vi "GCDiode.vi"(2 "Run uninterrupted?":bool, 3 "Device Category IN:":string(combo)="ATLAS18SS" caption="Device Category:", 4 "Batch No. IN:":string caption="Batch No.:", 5 "Wafer No. IN:":string caption="Wafer No.:", 6 "DB Serial No. IN:":string caption="DB Serial No.:") -> (0 "Done!":bool)   [LabVIEW 2013]
doc: "Performs measurements on gate-controlled diodes on sensor halfmoons according to ATLAS ITk QA Specifications."
uses:
  InstrControl/SupplyControl/SupplyControl.lvclass
  general_VIs/globals/QC_MeasurementSetup.vi
  general_VIs/globals/QC_RunInformation.vi
  InstrControl/InstrumentSetup.vi
  InstrControl/ArduinoControl/ArduinoControl.lvclass
  <vilib>/Analysis/NI_AALBase.lvlib
  InstrControl/InstrControl.lvclass
panel:
  out "Tab Control 2":enum32{"GCD Setup", "GCD Scan"}(tab)
  in  "Bias voltage [V]":dbl=5.0
  in  "Set current limit?":bool
  in  "Current Limit [µA]":dbl=1000.0 min=0.0001 format="%.3f"
  in  "Measurement Configurations":bool
  in  "Initial volts [V] IN":dbl=-10.0 caption="Initial volts [V]"
  in  "Final volts [V] IN":dbl=20.0 caption="Final volts [V]"
  in  "step [V] IN":dbl=0.5 caption="step [V]" format="%.1f"
  in  "step interval [s] IN":i32=1 caption="step interval [s]"
  in  "Continue":bool
  in  "Quit":bool
  out "Bias volts [V]":dbl=5.0 format="%.1f"
  out "RH":dbl[](array[numeric]) caption="RH [%]" format="%#.2f"
  out "Temp.":dbl[](array[numeric]) caption="Temp. [°C]" format="%#.2f"
  out "Current":dbl[](array[numeric]) caption="Current [nA]"
  out "Volts":dbl[](array[numeric]) caption="Volts [V]"
  out "step interval [s]":i32=1
  out "step [V]":dbl=0.5 format="%.1f"
  out "Final volts [V]":dbl=20.0 format="%.1f"
  out "Initial volts [V]":dbl=-10.0 format="%.1f"
  out "Igraph":cluster{dbl[], dbl[]}(graph)
  in  "Scales":T1(ring)
  in  "Iscale":enum16{"nanoAmps", "microAmps", "milliAmps"}(ring)
  out "positive ramp?":bool
  out "Tab Control":enum32{"GCD Setup", "GCD Scan"}(tab)
  in  "Test SMU":string(combo)="Keithley 2410"
  in  "Hardware Configurations":bool
  in  "User:":string(combo)="Christoph"
  in  "Bias Supply":string(combo)="Keithley 6517"
  in  "Temperature":enum16{"Read Arduino", "Enter manually"}(ring)=enum."Enter manually"
  in  "Manufacturer:":string(combo)="Hamamatsu"
  in  "abort":bool
  out "Device Category:":string
  out "DB Serial No.:":string
  out "Current Volts:":dbl format="%.2f"
  in  "quit (no save)":bool
  in  "Quit & Save":bool
  out "Bias On/Off:":bool
  out "STATUS 1":string
  out "Initiated:":string
  out "Sensor No.:":string
  out "No of steps":u32
  out "Current reading No.":u32
  out "Last reading at:":string
  # "University of\nCambridge"
  # "Strip Sensor QA: Gate-controlled Diode"
  # "Vertical Scale:"
  # "Measurement Configuration"
  # "IV Scan parameters:"
  # "Last 3 readings:"
  # "n-2"
  # "n-1"
  # "n"
  # "DUT Description"
  # "Hardware"
  # "DUT & Test Description:"
  # "Current status:"
  # "Rdg No:"
  # "out of"
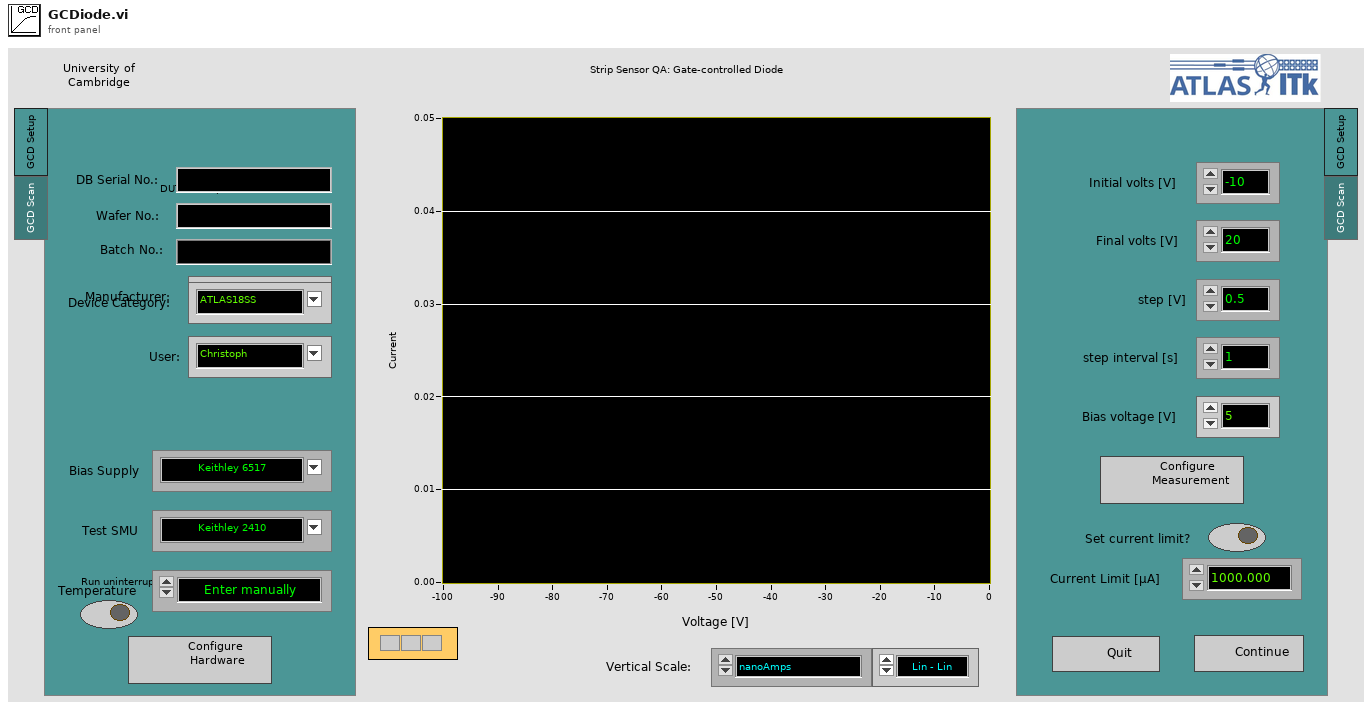
[diagram p1: front panel]
types:
  T1 = enum16{"Lin - Lin", "Log - Lin", "Lin - Log", "Log - log"}
  T2 = enum16{"Supply", "LCR", "Multimeter", "Switching"}
  T3 = enum16{"Reset", "Read Array", "Read Element", "Write Element", "Write Array", "Add Element", "Add Array"}
  T4 = cluster{"Institute":string, "Manufacturers":string[], "Devices":string[], "Serialnumbers Lookup DB":string, "Data directory":string, "Backup & screenshot directory":string, "List of known users":string[], "Measurement switch not used":bool, "Measurement Switch":string, "DUT Switch":string, "Rseries IV [MOhm]":string, "Rshunt IV [MOhm]":string, "Rseries CV [MOhm]":string, "DC blocking Cap [µF]":string, "Rseries LCR [MOhm]":string, "Rseries stability [MOhm]":string, "Rshunt stability [MOhm]":string, "Rseries striptest bias [MOhm]":string, "Rseries strip pinhole [MOhm]":string}
  T5 = cluster{"Sensor Serial No.:":string, "Wafer:":string, "Batch:":string, "Manufacturer:":string, "Device Category:":string, "Database Serial No.:":string, "Date Initiated:":string, "Time Initiated:":string, "Test":string, "Probeplan used:":string, "End of Run comment:":string, "User:":string, "Vbias SMU":string, "LCR":string, "Test SMU":string, "Test DMM":string}
  T6 = cluster{"Bias Supply":refnum<class "SupplyControl.lvclass">, "SMU":refnum<class "SupplyControl.lvclass">, "Arduino":refnum<class "ArduinoControl.lvclass">, "Initial Voltage [V]":dbl, "Final Voltage [V]":dbl, "Step Size [V]":dbl, "Step Interval [s]":i32, "Number Of Steps":u32, "Ramp down steps [V]":dbl, "Ramp down Interval [s]":i32, "Bias Voltage [V]":dbl, "Set Current Limit?":bool, "Current Limit [µA]":dbl, "Temperature Readout":enum16{"Read Arduino", "Enter manually"}, "Bias Supply Name":string, "SMU Name":string}
  T7 = cluster{"VISA address":refnum<visa-resource-name>, "T sensor":enum16{"SHT", "DS"}, "Arduino":refnum<class "ArduinoControl.lvclass">}
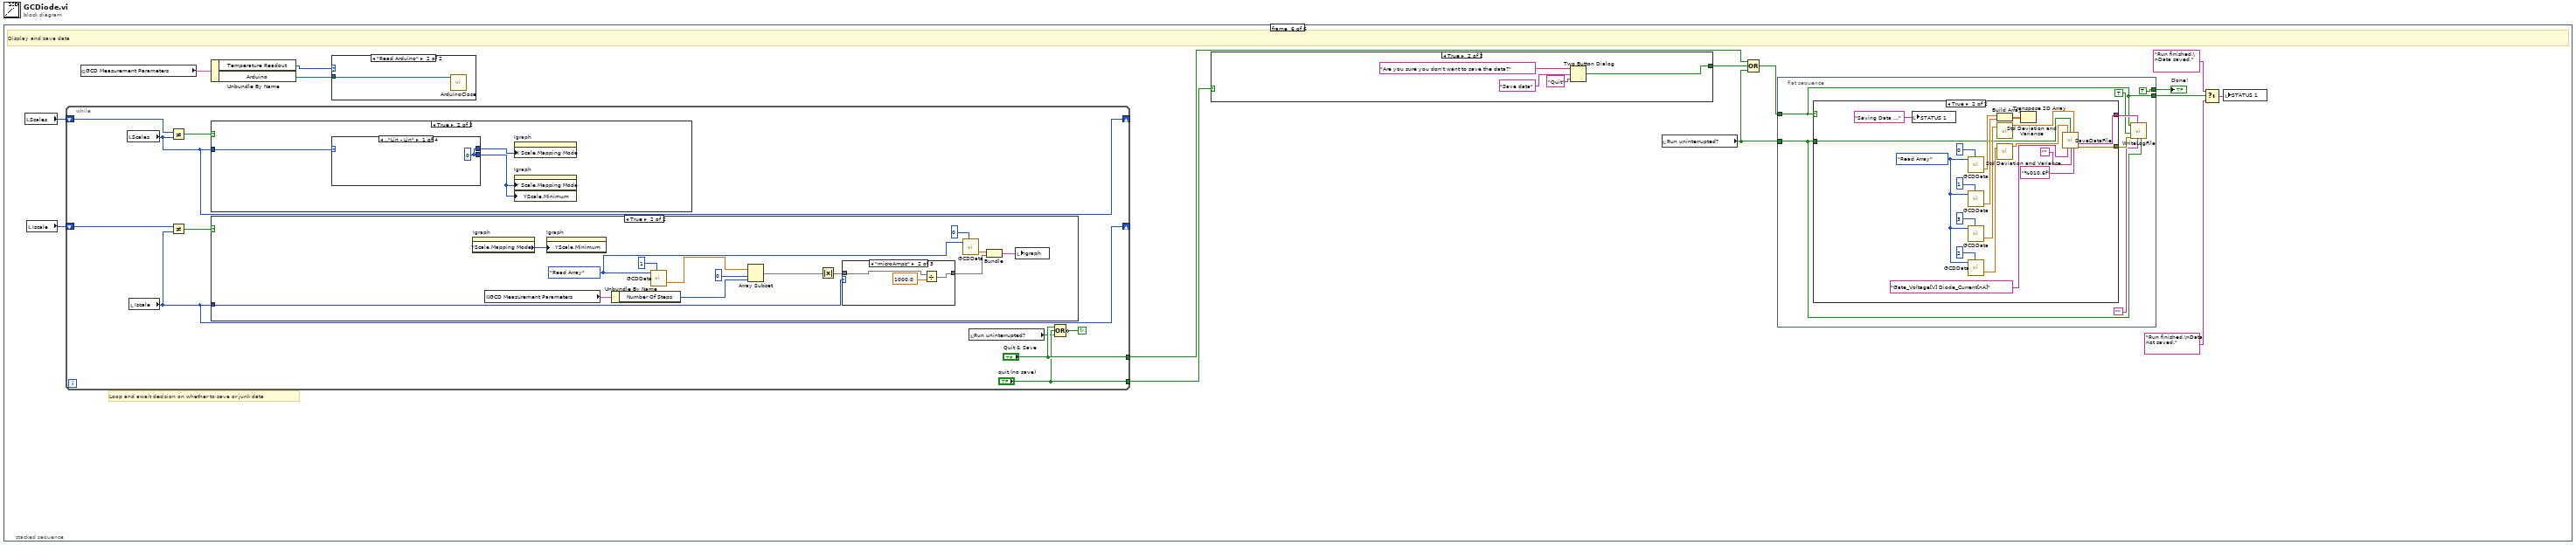
[diagram p0: block diagram]
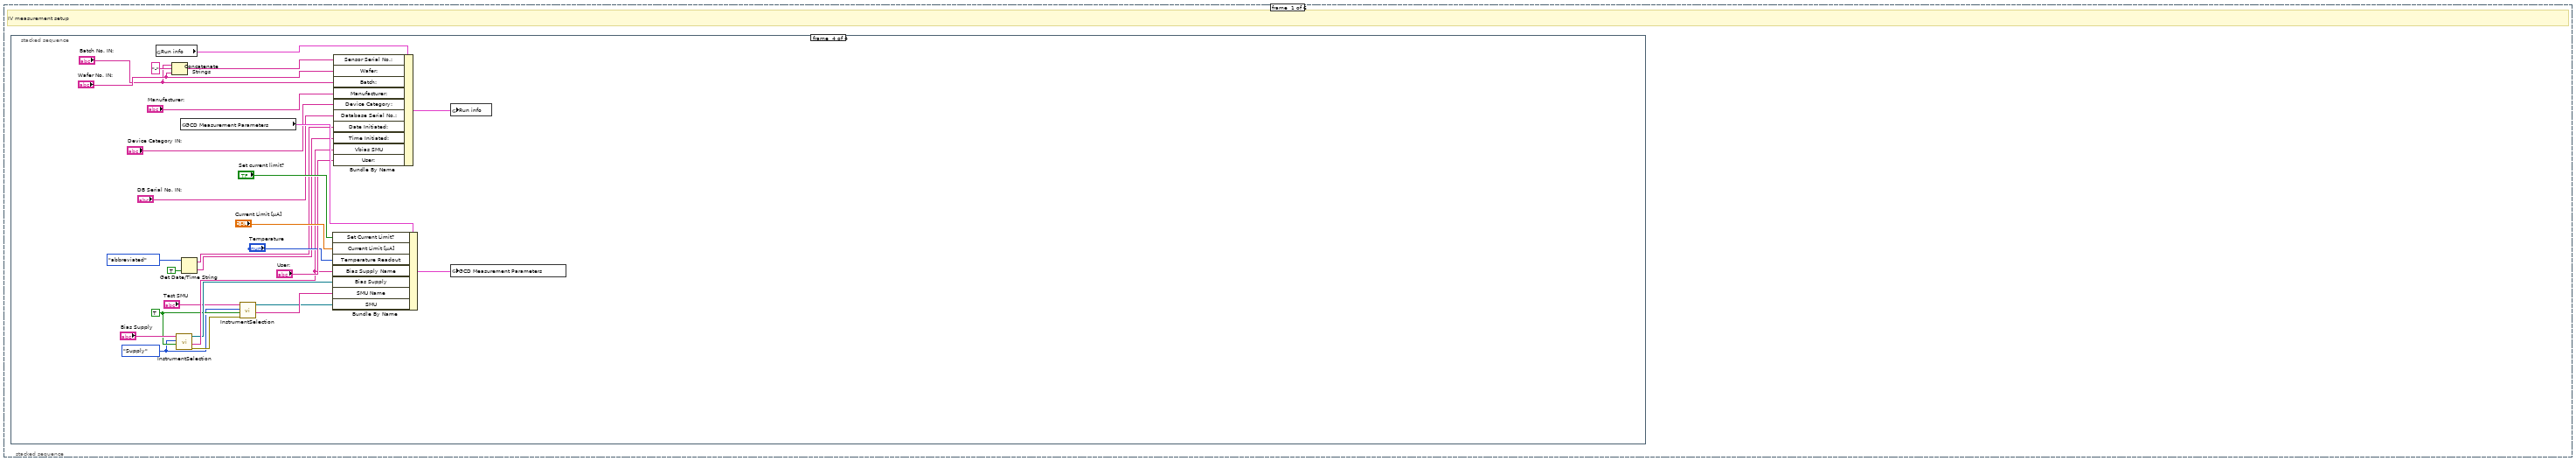
[diagram p2: hidden frame]
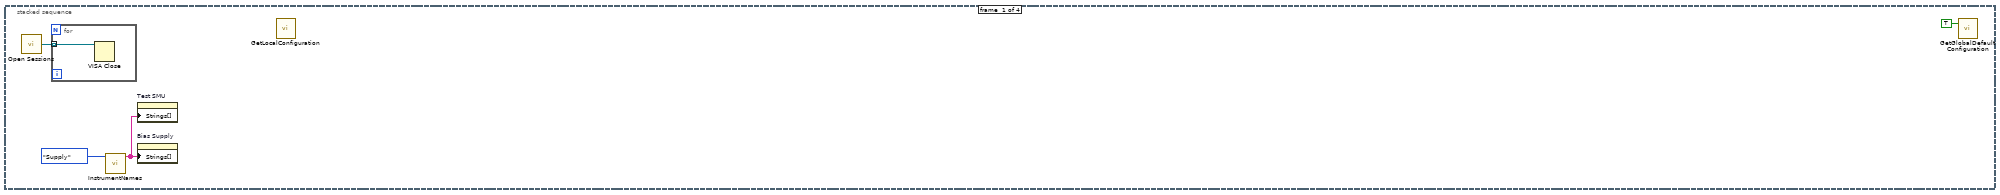
[diagram p3: hidden frame]
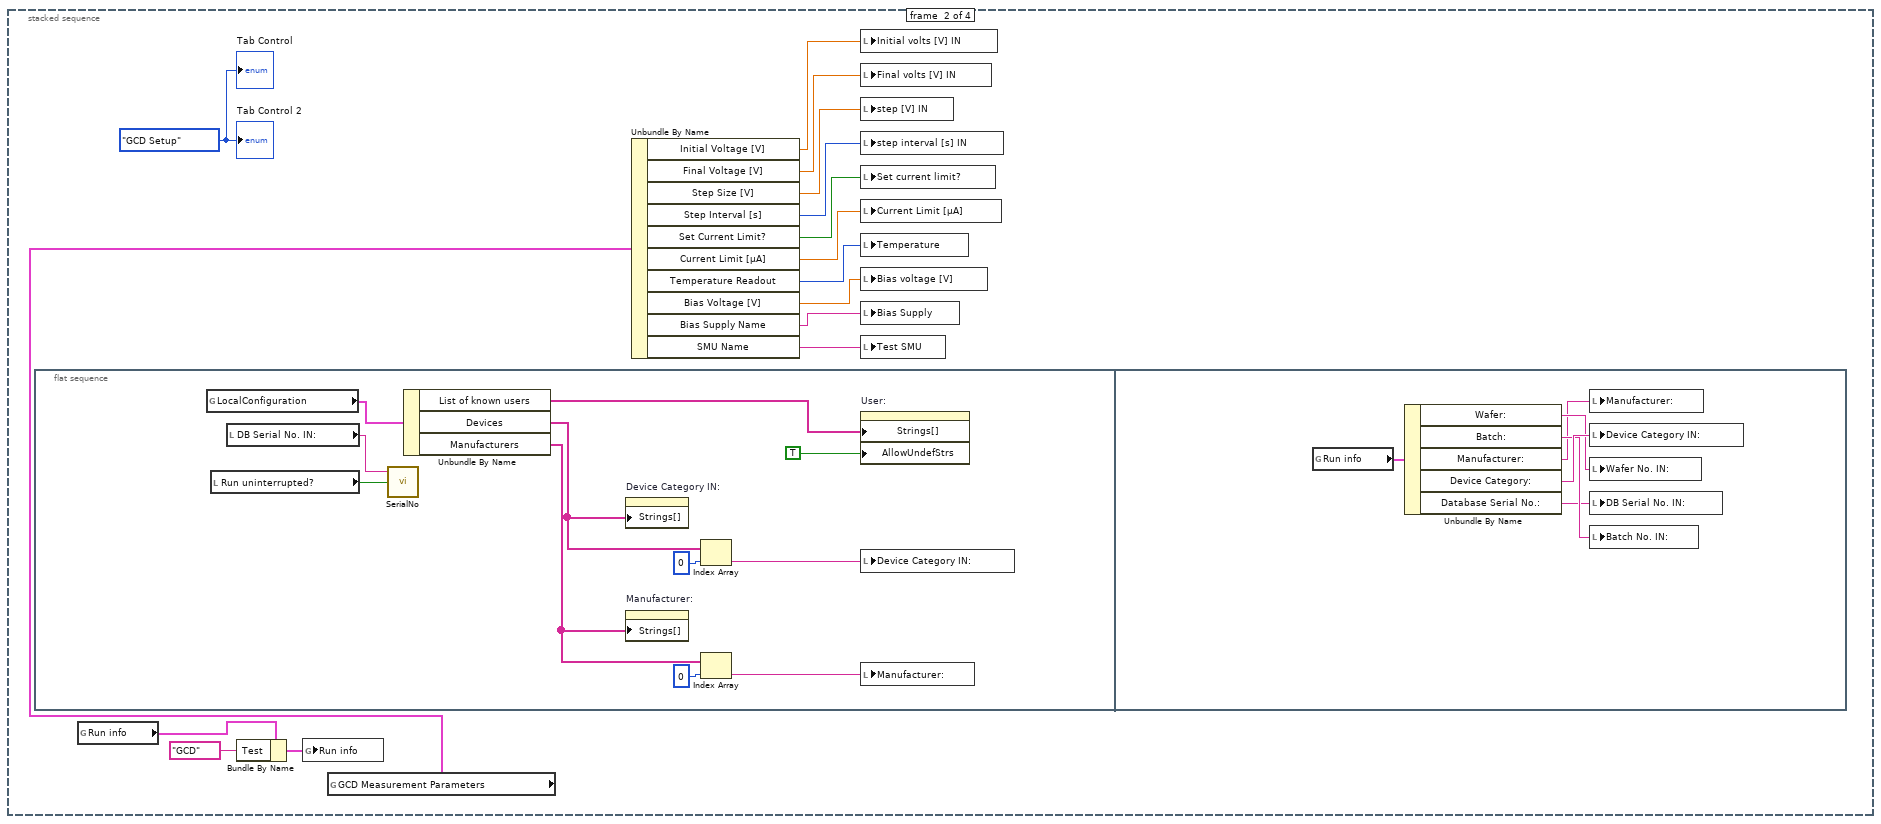
[diagram p4: hidden frame]
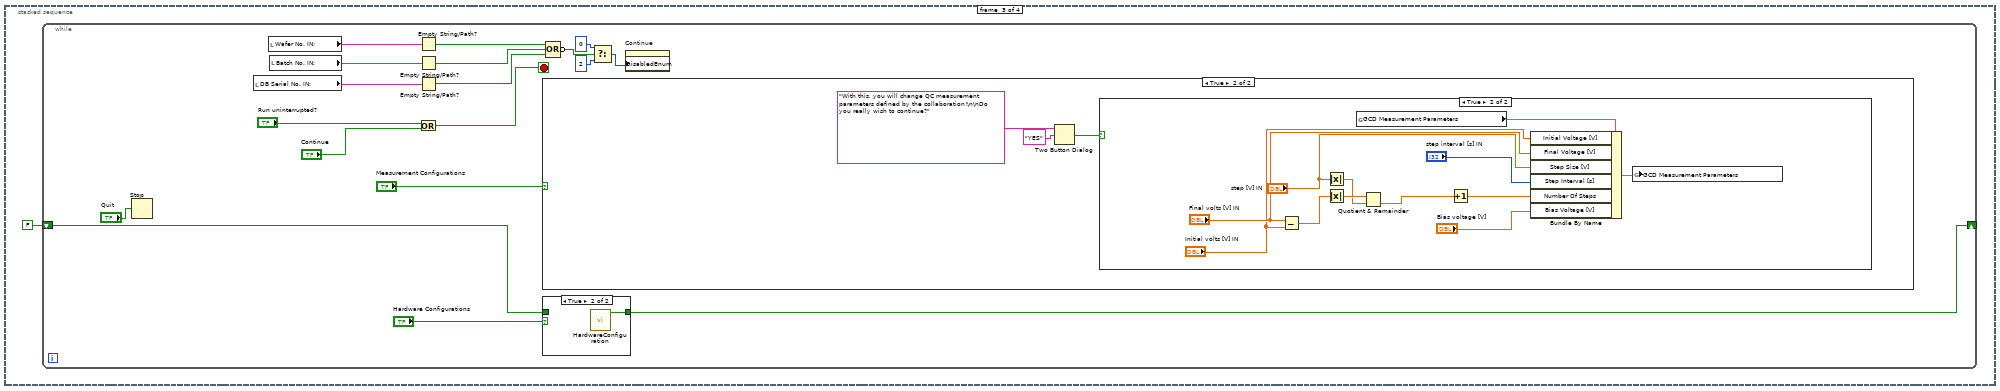
[diagram p5: hidden frame]
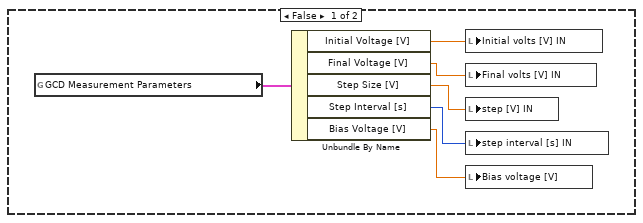
[diagram p7: hidden frame]
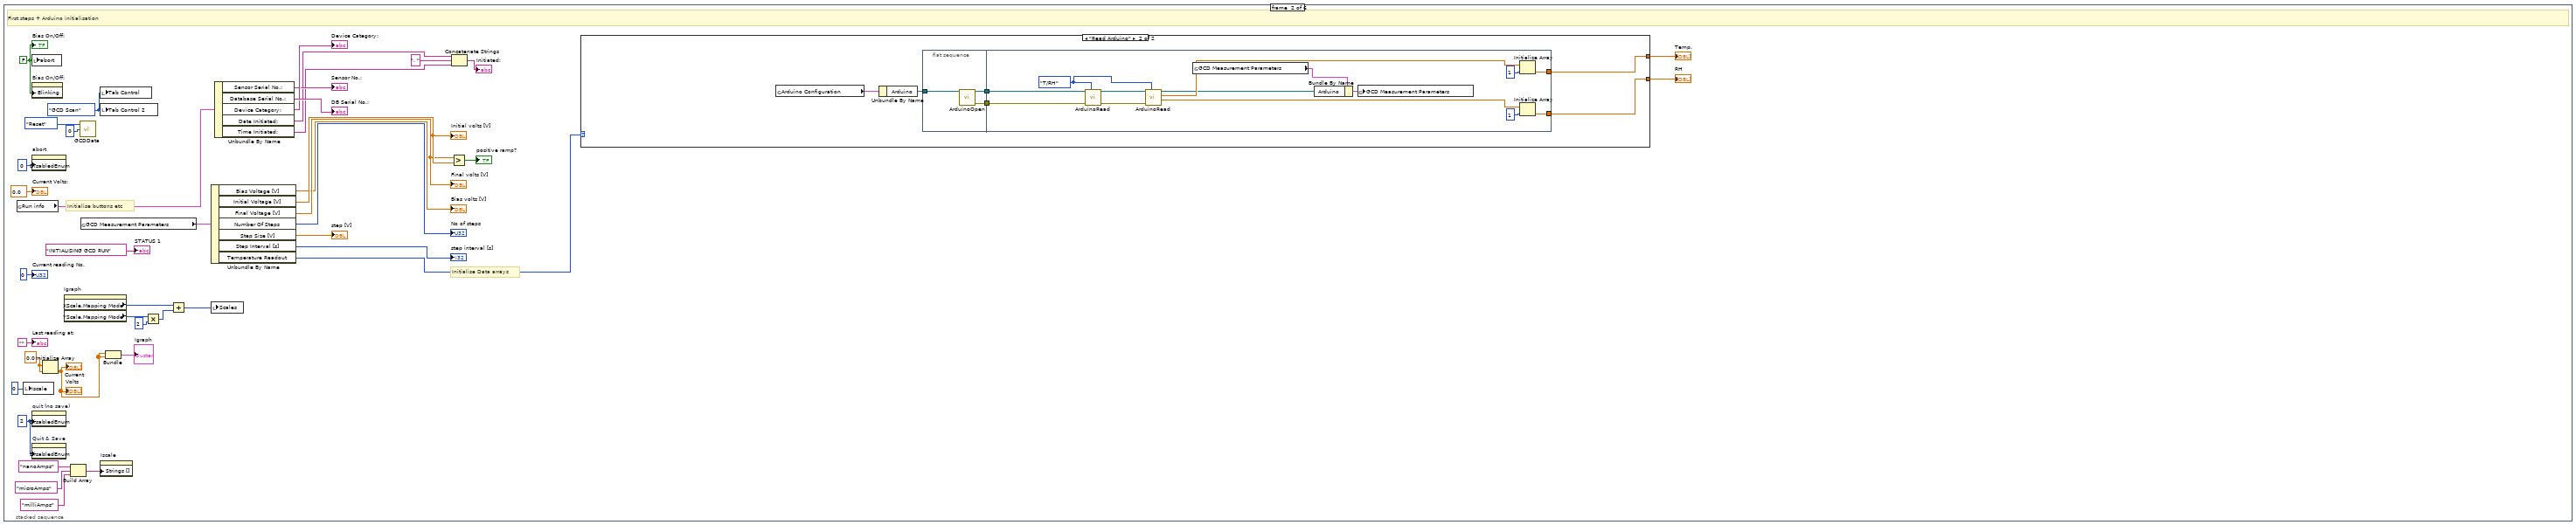
[diagram p9: hidden frame]
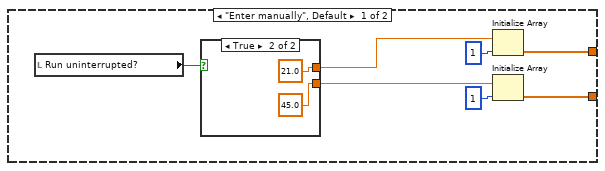
[diagram p10: hidden frame]
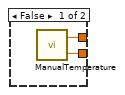
[diagram p11: hidden frame]
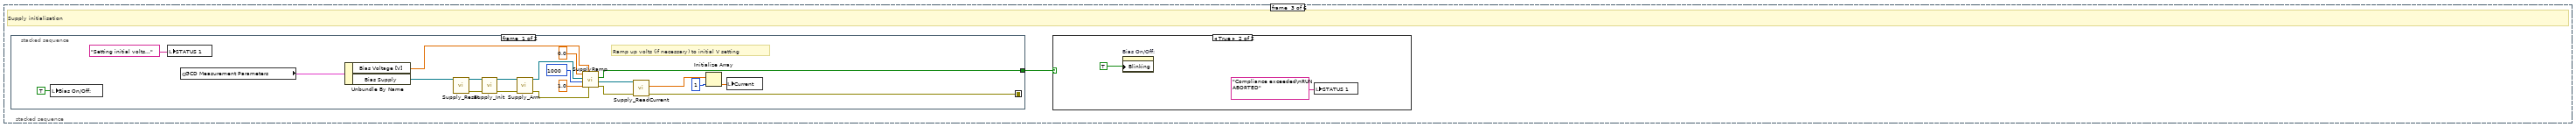
[diagram p12: hidden frame]
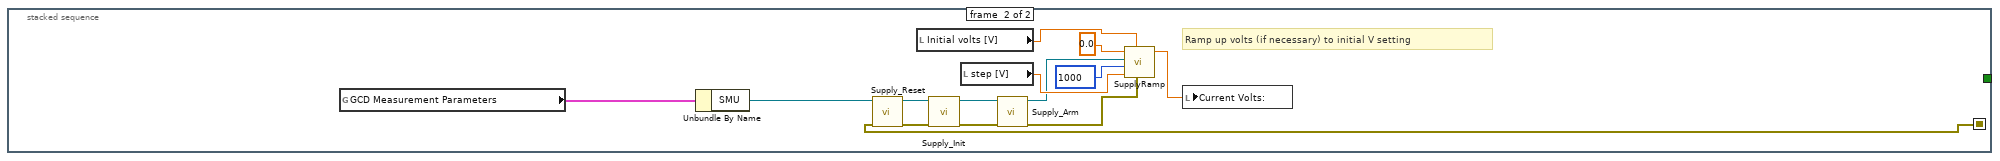
[diagram p13: hidden frame]
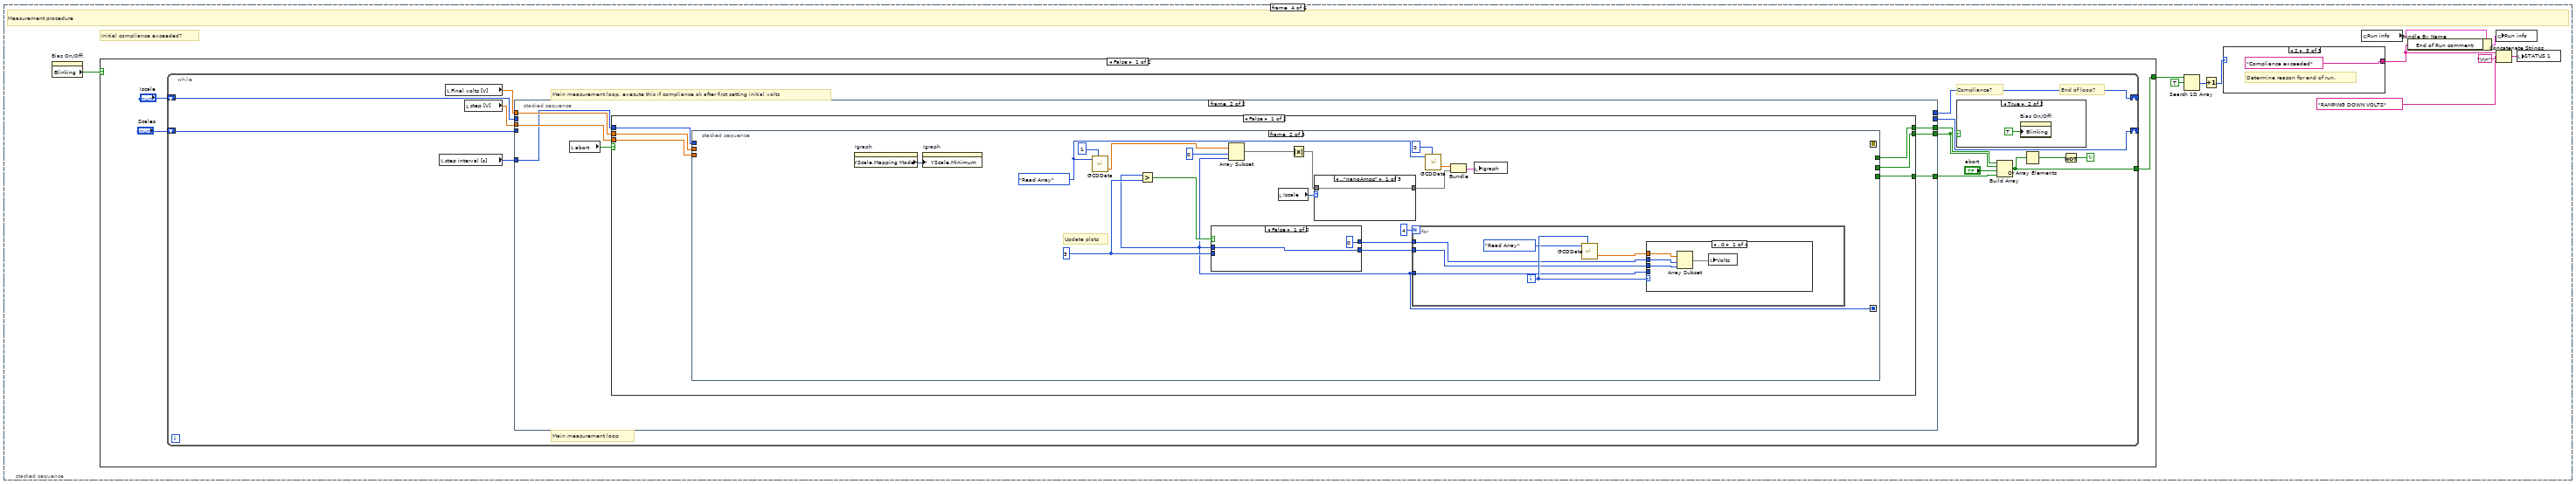
[diagram p15: hidden frame]
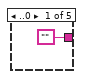
[diagram p16: hidden frame]
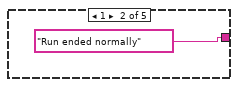
[diagram p17: hidden frame]
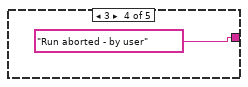
[diagram p18: hidden frame]
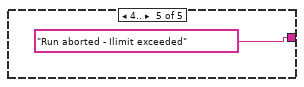
[diagram p19: hidden frame]
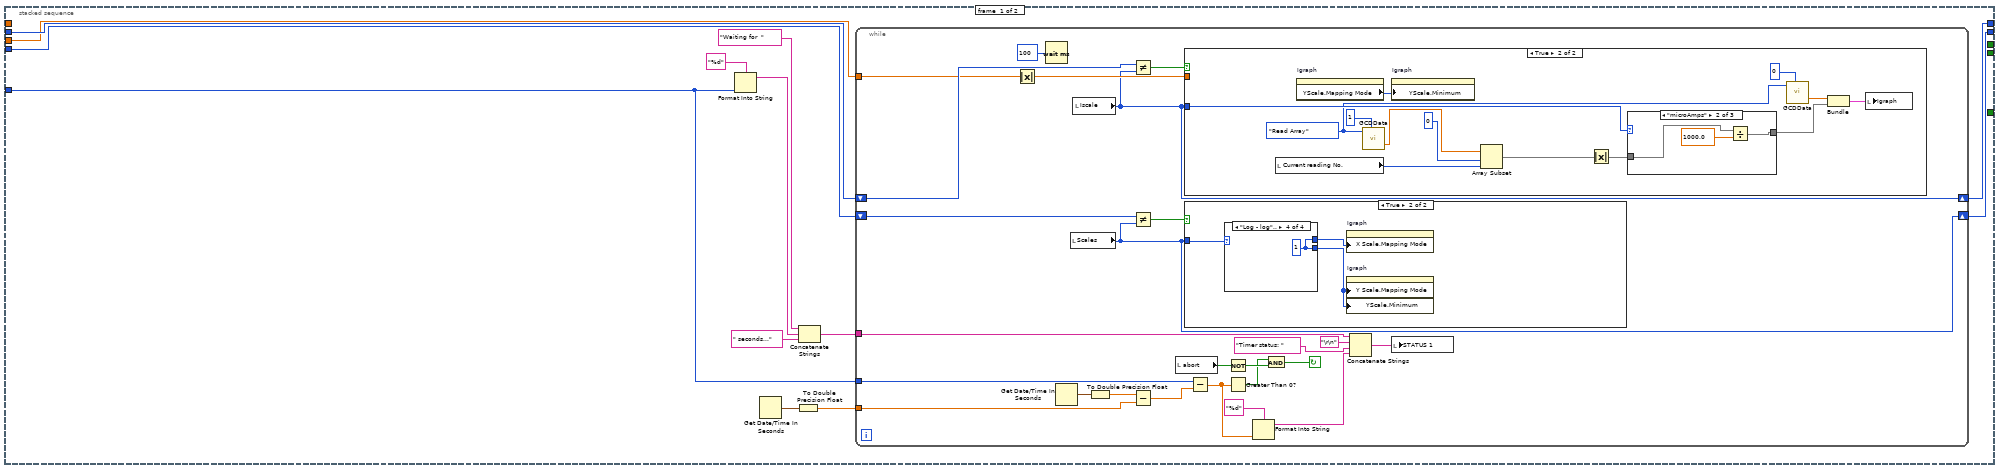
[diagram p20: hidden frame]
diagram:
  n1 = stacked-sequence {
    frame #0 {
      # "IV measurement setup"
      n2 = stacked-sequence {
        frame #0 {
          n3 = call <vilib>:"Open Sessions.vi"() -> ("Array of Refnums"=w2:refnum<visa-resource-name>[])  [unwired: 2 in]
          n4 = for {
            tunnel: w2 -> [w5] mode=indexing
            n5 = VISA Close(VISA resource name=w5) -> ()  [unwired: 1 in, 1 out]
          }
          n6 = call "InstrumentNames.vi"("Instrument type"=T2."Supply") -> ("Instrument names"=w1:string[])  [unwired: 9 in, 1 out]
          n7 = property on="Test SMU" class="CmbBox"("Strings[]"=w1) -> ()  [unwired: 2 in, 2 out]
          n8 = property on="Bias Supply" class="CmbBox"("Strings[]"=w1) -> ()  [unwired: 2 in, 2 out]
          n9 = call "GetLocalConfiguration.vi"() -> ()  [unwired: 3 in, 1 out]
          n10 = call "GetGlobalDefaultConfiguration.vi"("Read defaults?"=TRUE) -> ()  [unwired: 3 in]
        }
        frame #1 {
          w9 = enum32{"GCD Setup", "GCD Scan"}."GCD Setup" ("Tab Control")
          n11 = flat-sequence {
            frame #0 {
              n12 = global read "QC_RunInformation.vi" "LocalConfiguration"() -> (w23:T4)
              n13 = local read "Run uninterrupted?"() -> (w22:bool)
              n14 = local read "DB Serial No. IN:"() -> (w21:string)
              n15 = call "SerialNo.vi"("DB serial number IN"=w21, "Run uninterrupted?"=w22) -> ()  [unwired: 6 in, 2 out]
              n16 = Unbundle By Name(w23) -> ("List of known users"=w24:string[], "Devices"=w27:string[], "Manufacturers"=w29:string[])
              n17 = property on="Device Category IN:" class="CmbBox"("Strings[]"=w27) -> ()  [unwired: 2 in, 2 out]
              n18 = property on="Manufacturer:" class="CmbBox"("Strings[]"=w29) -> ()  [unwired: 2 in, 2 out]
              n19 = Index Array(array=w27, index=0) -> (element=w31:string)
              n20 = Index Array(array=w29, index=0) -> (element=w30:string)
              n21 = property on="User:" class="CmbBox"("Strings[]"=w24, "AllowUndefStrs"=TRUE) -> ()  [unwired: 2 in, 2 out]
              n22 = local write "Device Category IN:"(w31) -> ()
              n23 = local write "Manufacturer:"(w30) -> ()
            }
            frame #1 {
              n24 = global read "QC_RunInformation.vi" "Run info"() -> (w32:T5)
              n25 = Unbundle By Name(w32) -> ("Wafer:"=w36:string, "Batch:"=w35:string, "Manufacturer:"=w34:string, "Device Category:"=w37:string, "Database Serial No.:"=w33:string)
              n26 = local write "Manufacturer:"(w34) -> ()
              n27 = local write "Device Category IN:"(w37) -> ()
              n28 = local write "Wafer No. IN:"(w36) -> ()
              n29 = local write "DB Serial No. IN:"(w33) -> ()
              n30 = local write "Batch No. IN:"(w35) -> ()
            }
          }
          n31 = global read "QC_RunInformation.vi" "Run info"() -> (w16:T5)
          n32 = Bundle By Name(cluster=w16, "Test"="GCD") -> (w15:T5)
          n33 = global write "QC_RunInformation.vi" "Run info"(w15) -> ()
          n34 = global read "QC_MeasurementSetup.vi" "GCD Measurement Parameters"() -> (w19:T6)
          n35 = Unbundle By Name(w19) -> ("Initial Voltage [V]"=w13:dbl, "Final Voltage [V]"=w12:dbl, "Step Size [V]"=w11:dbl, "Step Interval [s]"=w14:i32, "Set Current Limit?"=w18:bool, "Current Limit [µA]"=w17:dbl, "Temperature Readout"=w20:enum16{"Read Arduino", "Enter manually"}, "Bias Voltage [V]"=w10:dbl, "Bias Supply Name"=w7:string, "SMU Name"=w6:string)
          n36 = local write "Initial volts [V] IN"(w13) -> ()
          n37 = local write "Final volts [V] IN"(w12) -> ()
          n38 = local write "step [V] IN"(w11) -> ()
          n39 = local write "step interval [s] IN"(w14) -> ()
          n40 = local write "Set current limit?"(w18) -> ()
          n41 = local write "Current Limit [µA]"(w17) -> ()
          n42 = local write "Temperature"(w20) -> ()
          n43 = local write "Bias voltage [V]"(w10) -> ()
          n44 = local write "Bias Supply"(w7) -> ()
          n45 = local write "Test SMU"(w6) -> ()
          "Tab Control" <- w9
          "Tab Control 2" <- w9
        }
        frame #2 {
          n46 = while {
            shift-right: [w46] -> _
            shift-left: FALSE -> [w45]
            stop <- w42 stop-if-true
            n47 = Stop(stop? (T)="Quit") -> ()
            n48 = local read "DB Serial No. IN:"() -> (w40:string)
            n49 = local read "Wafer No. IN:"() -> (w55:string)
            n50 = local read "Batch No. IN:"() -> (w48:string)
            n51 = Empty String/Path?(string/path=w55) -> (empty?=w54:bool)
            n52 = Empty String/Path?(string/path=w48) -> (empty?=w47:bool)
            n53 = Empty String/Path?(string/path=w40) -> (empty?=w39:bool)
            n54 = Or(x="Run uninterrupted?", y="Continue") -> (x .or. y?=w42:bool)
            n55 = case shown="True" "Measurement Configurations" {
              frame False {
              }
              frame True {
                n56 = Two Button Dialog(message="With this, you will change QC measurement parameters defined by the collaboration!\n\nDo you really wish to continue?", 2:"YES") -> (T button?=w57:bool)  [unwired: 1 in]
                n57 = case shown="True" w57 {
                  frame False {
                    n58 = global read "QC_MeasurementSetup.vi" "GCD Measurement Parameters"() -> (w65:T6)
                    n59 = Unbundle By Name(w65) -> ("Initial Voltage [V]"=w63:dbl, "Final Voltage [V]"=w64:dbl, "Step Size [V]"=w62:dbl, "Step Interval [s]"=w61:i32, "Bias Voltage [V]"=w60:dbl)
                    n60 = local write "Initial volts [V] IN"(w63) -> ()
                    n61 = local write "Final volts [V] IN"(w64) -> ()
                    n62 = local write "step [V] IN"(w62) -> ()
                    n63 = local write "step interval [s] IN"(w61) -> ()
                    n64 = local write "Bias voltage [V]"(w60) -> ()
                  }
                  frame True {
                    n65 = Subtract(x="Final volts [V] IN", y="Initial volts [V] IN") -> (x-y=w71:dbl)
                    n66 = Absolute Value(x="step [V] IN") -> (abs(x)=w72:dbl)
                    n67 = Absolute Value(x=w71) -> (abs(x)=w73:dbl)
                    n68 = global read "QC_MeasurementSetup.vi" "GCD Measurement Parameters"() -> (w77:T6)
                    n69 = Quotient & Remainder(x=w73, y=w72) -> (floor(x/y)=w69:dbl)  [unwired: 1 out]
                    n70 = Increment(x=w69) -> (x+1=w68:dbl)
                    n71 = Bundle By Name(cluster=w77, "Initial Voltage [V]"="Initial volts [V] IN", "Final Voltage [V]"="Final volts [V] IN", "Step Size [V]"="step [V] IN", "Step Interval [s]"="step interval [s] IN", "Number Of Steps"=w68, "Bias Voltage [V]"="Bias voltage [V]") -> (w74:T6)
                    n72 = global write "QC_MeasurementSetup.vi" "GCD Measurement Parameters"(w74) -> ()
                  }
                }
              }
            }
            n73 = case shown="True" "Hardware Configurations" {
              tunnel: [w78 w79] -> w46
              tunnel: w45 -> [w78 _]
              frame False {
              }
              frame True {
                n74 = call "HardwareConfiguration.vi"() -> ("configured?"=w79:bool)  [unwired: 11 in]
              }
            }
            n75 = Compound Arithmetic op=OR(w54, w47, w39) -> (invert w53:bool)
            n76 = Select(t=0, s=w53, f=2) -> (s? t:f=w50:i32)
            n77 = property on="Continue" class="Bool"("DisabledEnum"=w50) -> ()  [unwired: 2 in, 2 out]
          }
        }
        frame #3 {
          w85 = TRUE
          w80 = T2."Supply" ("Instrument type")
          n78 = global read "QC_RunInformation.vi" "Run info"() -> (w86:T5)
          n79 = Concatenate Strings("Batch No. IN:", "-", "Wafer No. IN:") -> (w87:string)
          n80 = call "InstrumentSelection.vi"("Verify GPIB address"=w85, "Instrument type"=w80, "Instrument name IN"="Bias Supply") -> ("error out"=w83:errorcluster, "Instrument name OUT"=w96:string, "Supply"=w95:refnum<class "SupplyControl.lvclass">)  [unwired: 3 in, 3 out]
          n81 = global read "QC_MeasurementSetup.vi" "GCD Measurement Parameters"() -> (w106:T6)
          n82 = Get Date/Time String(date format (0)=enum16{"short", "long", "abbreviated"}."abbreviated", want seconds? (F)=TRUE) -> (date string=w92:string, time string=w91:string)  [unwired: 1 in]
          n83 = call "InstrumentSelection.vi"("error in (no error)"=w83, "Verify GPIB address"=w85, "Instrument type"=w80, "Instrument name IN"="Test SMU") -> ("Instrument name OUT"=w82:string, "Supply"=w81:refnum<class "SupplyControl.lvclass">)  [unwired: 2 in, 4 out]
          n84 = Bundle By Name(cluster=w106, "Set Current Limit?"="Set current limit?", "Current Limit [µA]"="Current Limit [µA]", "Temperature Readout"="Temperature", "Bias Supply Name"=w96, "Bias Supply"=w95, "SMU Name"=w82, "SMU"=w81) -> (w107:T6)
          n85 = Bundle By Name(cluster=w86, "Sensor Serial No.:"=w87, "Wafer:"="Wafer No. IN:", "Batch:"="Batch No. IN:", "Manufacturer:"="Manufacturer:", "Device Category:"="Device Category IN:", "Database Serial No.:"="DB Serial No. IN:", "Date Initiated:"=w92, "Time Initiated:"=w91, "Vbias SMU"=w96, "User:"="User:") -> (w101:T5)
          n86 = global write "QC_RunInformation.vi" "Run info"(w101) -> ()
          n87 = global write "QC_MeasurementSetup.vi" "GCD Measurement Parameters"(w107) -> ()
        }
      }
    }
    frame #1 {
      w109 = enum32{"GCD Setup", "GCD Scan"}."GCD Scan" ("Tab Control")
      w132 = 2
      w139 = 0.0
      w131 = FALSE ("Visible")
      # "Initialise buttons etc"
      # "Initialise Data arrays"
      # "First steps + Arduino initialisation"
      n88 = global read "QC_RunInformation.vi" "Run info"() -> (w148:T5)
      n89 = local write "Iscale"(u16 0 ("Scale")) -> ()
      n90 = local write "abort"(w131) -> ()
      n91 = property on="Bias On/Off:" class="Bool (strict)"("Blinking"=w131) -> ()  [unwired: 2 in, 2 out]
      n92 = property on="abort" class="Bool (strict)"("DisabledEnum"=0) -> ()  [unwired: 2 in, 2 out]
      n93 = property on="quit (no save)" class="Bool"("DisabledEnum"=w132) -> ()  [unwired: 2 in, 2 out]
      n94 = property on="Quit & Save" class="Bool"("DisabledEnum"=w132) -> ()  [unwired: 2 in, 2 out]
      n95 = Initialize Array(w139, w139) -> (w117:dbl[])
      "Volts" <- w117
      "Current" <- w117
      n96 = property on="Igraph" class="XYGraph (strict)"() -> ("XScale.Mapping Mode"=w124:u8, "YScale.Mapping Mode"=w123:u8)  [unwired: 2 in, 2 out]
      n97 = Build Array("nanoAmps", "microAmps", "milliAmps") -> (w145:string[])
      n98 = call "GCDData.vi"("Action"=T3."Reset", "Array Size / Index"=0) -> ()  [unwired: 3 in, 2 out]
      n99 = global read "QC_MeasurementSetup.vi" "GCD Measurement Parameters"() -> (w120:T6)
      n100 = local write "Tab Control"(w109) -> ()
      n101 = local write "Tab Control 2"(w109) -> ()
      n102 = property on="Iscale" class="Enum (strict)"("Strings []"=w145) -> ()  [unwired: 2 in, 2 out]
      n103 = Bundle(w117, w117) -> (→"Igraph":cluster{dbl[], dbl[]})  [unwired: 1 in]
      n104 = Multiply(x=w123, y=2) -> (x*y=w126:i32)
      n105 = Add(x=w124, y=w126) -> (x+y=w122:i32)
      n106 = Unbundle By Name(w120) -> ("Bias Voltage [V]"=→"Bias volts [V]":dbl, "Initial Voltage [V]"=w130:dbl, "Final Voltage [V]"=w129:dbl, "Number Of Steps"=→"No of steps":u32, "Step Size [V]"=→"step [V]":dbl, "Step Interval [s]"=→"step interval [s]":i32, "Temperature Readout"=w133:enum16{"Read Arduino", "Enter manually"})
      "Initial volts [V]" <- w130
      "Final volts [V]" <- w129
      n107 = local write "Scales"(w122) -> ()
      n108 = Unbundle By Name(w148) -> ("Sensor Serial No.:"=→"Sensor No.:":string, "Database Serial No.:"=→"DB Serial No.:":string, "Device Category:"=→"Device Category:":string, "Date Initiated:"=w115:string, "Time Initiated:"=w114:string)
      n109 = Greater?(x=w129, y=w130) -> (0:→"positive ramp?":bool)
      n110 = Concatenate Strings(w115, ", ", w114) -> (→"Initiated:":string)
      n111 = case shown="\"Read Arduino\"" w133 {
        tunnel: [w156 w166] -> w136
        tunnel: [w155 w165] -> w121
        frame "Enter manually", Default {
          n112 = local read "Run uninterrupted?"() -> (w150:bool)
          n113 = case shown="True" w150 {
            tunnel: [w158 21.0] -> w154
            tunnel: [w157 45.0] -> w151
            frame False {
              n114 = call "ManualTemperature.vi"() -> ("Humidity [%] out"=w157:dbl, "Temperature [°C] out"=w158:dbl)
            }
            frame True {
            }
          }
          n115 = Initialize Array(w154, 1) -> (w156:dbl[])
          n116 = Initialize Array(w151, 1) -> (w155:dbl[])
        }
        frame "Read Arduino" {
          n117 = global read "InstrumentSetup.vi" "Arduino Configuration"() -> (w162:T7)
          n118 = Unbundle By Name(w162) -> ("Arduino"=w161:refnum<class "ArduinoControl.lvclass">)
          n119 = flat-sequence {
            tunnel: [w167] -> w164
            tunnel: [w169] -> w163
            tunnel: w161 -> [w168]
            tunnel: [w183] -> w166
            tunnel: [w180] -> w165
            tunnel: w164 -> [w174]
            tunnel: w163 -> [w173]
            frame #0 {
              n120 = call "ArduinoOpen.vi"("ArduinoControl in"=w168) -> ("error out"=w169:errorcluster, "ArduinoControl out"=w167:refnum<class "ArduinoControl.lvclass">)  [unwired: 9 in]
            }
            frame #1 {
              w170 = enum16{"T/RH", "Interlock", "Edgesense"}."T/RH" ("Arduino function")
              n121 = call "ArduinoRead.vi"("Arduino function"=w170, "error in (no error)"=w173, "ArduinoControl in"=w174) -> ("error out"=w172:errorcluster, "ArduinoControl out"=w171:refnum<class "ArduinoControl.lvclass">)  [unwired: 3 in, 4 out]
              n122 = call "ArduinoRead.vi"("Arduino function"=w170, "error in (no error)"=w172, "ArduinoControl in"=w171) -> ("rel. Humidity [%]"=w178:dbl, "Temperature [°C]"=w179:dbl, "ArduinoControl out"=w177:refnum<class "ArduinoControl.lvclass">)  [unwired: 3 in, 3 out]
              n123 = global read "QC_MeasurementSetup.vi" "GCD Measurement Parameters"() -> (w176:T6)
              n124 = Bundle By Name(cluster=w176, "Arduino"=w177) -> (w175:T6)
              n125 = global write "QC_MeasurementSetup.vi" "GCD Measurement Parameters"(w175) -> ()
              n126 = Initialize Array(w179, 1) -> (w183:dbl[])
              n127 = Initialize Array(w178, 1) -> (w180:dbl[])
            }
          }
        }
      }
      "Temp." <- w136
      "RH" <- w121
      "STATUS 1" <- "INITIALISING GCD RUN"
      "Bias On/Off:" <- w131
      "Last reading at:" <- ""
      "Current reading No." <- u32 0 ("Current reading No.")
      "Current Volts:" <- 0.0 ("Current Volts:")
    }
    frame #2 {
      # "Supply initialisation"
      n128 = stacked-sequence {
        seq-local: [w185 _] -> [_ w206]
        tunnel: [w188 _] -> w184
        frame #0 {
          # "Ramp up volts (if necessary) to initial V setting"
          n129 = local write "Bias On/Off:"(TRUE ("Compliance?")) -> ()
          n130 = local write "STATUS 1"("Setting initial volts..." ("STATUS 1")) -> ()
          n131 = global read "QC_MeasurementSetup.vi" "GCD Measurement Parameters"() -> (w201:T6)
          n132 = Unbundle By Name(w201) -> ("Bias Voltage [V]"=w187:dbl, "Bias Supply"=w198:refnum<class "SupplyControl.lvclass">)
          n133 = call-dynamic "Supply_Reset.vi"("SupplyControl in"=w198) -> ("error out"=w203:errorcluster, "SupplyControl out"=w205:refnum<class "SupplyControl.lvclass">)  [unwired: 9 in]
          n134 = call-dynamic "Supply_Init.vi"("error in (no error)"=w203, "SupplyControl in"=w205) -> ("error out"=w202:errorcluster, "SupplyControl out"=w204:refnum<class "SupplyControl.lvclass">)  [unwired: 8 in]
          n135 = call-dynamic "Supply_Arm.vi"("error in (no error)"=w202, "SupplyControl in"=w204) -> ("error out"=w194:errorcluster, "SupplyControl out"=w195:refnum<class "SupplyControl.lvclass">)  [unwired: 8 in]
          n136 = call "SupplyRamp.vi"("error in"=w194, "Requested Voltage"=w187, "Step Size"=1.0, "Step Delay"=1000, "Supply IN"=w195, "Starting Voltage"=0.0) -> ("error out"=w189:errorcluster, "Supply OUT"=w190:refnum<class "SupplyControl.lvclass">, "Compliance exceeded"=w188:bool)  [unwired: 2 in, 1 out]
          n137 = call-dynamic "Supply_ReadCurrent.vi"("error in (no error)"=w189, "SupplyControl in"=w190) -> ("error out"=w185:errorcluster, "Current in nA"=w192:dbl)  [unwired: 7 in, 1 out]
          n138 = Initialize Array(w192, 1) -> (w191:dbl[])
          n139 = local write "Current"(w191) -> ()
        }
        frame #1 {
          # "Ramp up volts (if necessary) to initial V setting"
          n140 = global read "QC_MeasurementSetup.vi" "GCD Measurement Parameters"() -> (w215:T6)
          n141 = Unbundle By Name(w215) -> ("SMU"=w214:refnum<class "SupplyControl.lvclass">)
          n142 = call-dynamic "Supply_Reset.vi"("error in (no error)"=w206, "SupplyControl in"=w214) -> ("error out"=w217:errorcluster, "SupplyControl out"=w219:refnum<class "SupplyControl.lvclass">)  [unwired: 8 in]
          n143 = local read "Initial volts [V]"() -> (w209:dbl)
          n144 = call-dynamic "Supply_Init.vi"("error in (no error)"=w217, "SupplyControl in"=w219) -> ("error out"=w216:errorcluster, "SupplyControl out"=w218:refnum<class "SupplyControl.lvclass">)  [unwired: 8 in]
          n145 = local read "step [V]"() -> (w210:dbl)
          n146 = call-dynamic "Supply_Arm.vi"("error in (no error)"=w216, "SupplyControl in"=w218) -> ("error out"=w207:errorcluster, "SupplyControl out"=w208:refnum<class "SupplyControl.lvclass">)  [unwired: 8 in]
          n147 = call "SupplyRamp.vi"("error in"=w207, "Requested Voltage"=w209, "Step Size"=w210, "Step Delay"=1000, "Supply IN"=w208, "Starting Voltage"=0.0) -> ("Current Voltage"=w213:dbl)  [unwired: 2 in, 3 out]
          n148 = local write "Current Volts:"(w213) -> ()
        }
      }
      n149 = case shown="True" w184 {
        frame False {
        }
        frame True {
          n150 = property on="Bias On/Off:" class="Bool (strict)"("Blinking"=TRUE) -> ()  [unwired: 2 in, 2 out]
          n151 = local write "STATUS 1"("Compliance exceeded\nRUN ABORTED") -> ()
        }
      }
    }
    frame #3 {
      # "Initial compliance exceeded?"
      # "Measurement procedure"
      n152 = property on="Bias On/Off:" class="Bool (strict)"() -> ("Blinking"=w232:bool)  [unwired: 2 in, 2 out]
      n153 = case shown="False" w232 {
        tunnel: [w240 w469] -> w231
        frame False {
          n154 = while {
            shift-left: "Iscale" -> [w250]
            shift-right: [w249] -> _
            shift-left: "Scales" -> [w251]
            shift-right: [w252] -> _
            tunnel: [w248] -> w240
            stop <- w253 continue-if-true
            # "Main measurement loop"
            # "End of loop?"
            # "Compliance?"
            # "Main measurement loop. execute this if compliance ok after first setting initial volts"
            n155 = local read "step interval [s]"() -> (w245:i32)
            n156 = local read "Final volts [V]"() -> (w246:dbl)
            n157 = local read "step [V]"() -> (w247:dbl)
            n158 = stacked-sequence {
              tunnel: [w267 _] -> w252
              tunnel: w247 -> [w264 w328]
              tunnel: [_ w327] -> w243
              tunnel: w246 -> [_ w326]
              tunnel: w245 -> [w255 w325]
              tunnel: [_ w324] -> w244
              tunnel: w251 -> [w266 _]
              tunnel: w250 -> [w265 _]
              tunnel: [w263 _] -> w249
              tunnel: [_ w322] -> w241
              frame #0 {
                n159 = Format Into String(format string="%d", w255) -> (resulting string=w260:string)  [unwired: 2 in, 1 out]
                n160 = Get Date/Time In Seconds() -> (seconds since 1Jan1904=w257:timestamp)
                n161 = To Double Precision Float(number=w257) -> (double precision float=w258:dbl)
                n162 = Concatenate Strings("Waiting for  ", w260, " seconds...") -> (w256:string)
                n163 = while {
                  tunnel: w264 -> [w276]
                  shift-left: w265 -> [w280]
                  shift-right: [w273] -> w263
                  shift-left: w266 -> [w281]
                  shift-right: [w282] -> w267
                  tunnel: w256 -> [w274]
                  tunnel: w255 -> [w286]
                  tunnel: w258 -> [w287]
                  stop <- w288 continue-if-true
                  n164 = Absolute Value(x=w276) -> (abs(x)=w275:dbl)
                  n165 = Wait (ms)(milliseconds to wait=u32 100) -> ()  [unwired: 1 out]
                  n166 = Get Date/Time In Seconds() -> (seconds since 1Jan1904=w272:timestamp)
                  n167 = local read "Scales"() -> (w282:T1)
                  n168 = local read "Iscale"() -> (w273:enum16{"nanoAmps", "microAmps", "milliAmps"})
                  n169 = To Double Precision Float(number=w272) -> (double precision float=w292:dbl)
                  n170 = Not Equal?(x=w280, y=w273) -> (x != y?=w271:bool)
                  n171 = Not Equal?(x=w281, y=w282) -> (x != y?=w283:bool)
                  n172 = Subtract(x=w292, y=w287) -> (x-y=w269:dbl)
                  n173 = local read "abort"() -> (w285:bool)
                  n174 = case shown="True" w271 {
                    tunnel: w275 -> [_ _]
                    tunnel: w273 -> [_ w300]
                    frame False {
                    }
                    frame True {
                      w294 = T3."Read Array" ("Action")
                      n175 = local read "Current reading No."() -> (w302:u32)
                      n176 = property on="Igraph" class="XYGraph (strict)"() -> ("YScale.Mapping Mode"=w296:u8)  [unwired: 2 in, 2 out]
                      n177 = call "GCDData.vi"("Action"=w294, "Array No."=u32 1 ("Action")) -> ("Array OUT"=w303:dbl[])  [unwired: 3 in, 1 out]
                      n178 = property on="Igraph" class="XYGraph (strict)"("YScale.Minimum"=w296) -> ()  [unwired: 2 in, 2 out]
                      n179 = Array Subset(array=w303, index=0, length=w302) -> (w299:dbl[])
                      n180 = Absolute Value(x=w299) -> (abs(x)=w298:dbl[])
                      n181 = case shown="\"microAmps\"" w300 {
                        tunnel: [w306 w307 w311] -> w305
                        tunnel: w298 -> [w306 w309 w312]
                        frame .."nanoAmps" {
                        }
                        frame "microAmps" {
                          n182 = Divide(x=w309, y=1000.0) -> (x/y=w307:dbl[])
                        }
                        frame "milliAmps".. {
                          n183 = Divide(x=w312, y=1000000.0) -> (x/y=w311:dbl[])
                        }
                      }
                      n184 = call "GCDData.vi"("Action"=w294, "Array No."=u32 0 ("Action")) -> ("Array OUT"=w293:dbl[])  [unwired: 3 in, 1 out]
                      n185 = Bundle("Array OUT"=w293, w305) -> (w301:cluster{"Array OUT":dbl[], dbl[]})  [unwired: 1 in]
                      n186 = local write "Igraph"(w301) -> ()
                    }
                  }
                  n187 = case shown="True" w283 {
                    tunnel: w282 -> [_ w315]
                    frame False {
                    }
                    frame True {
                      n188 = case shown="\"Log - log\".." w315 {
                        tunnel: [w316 1 0 w321] -> w314
                        tunnel: [w316 0 1 w321] -> w313
                        frame .."Lin - Lin" {
                          w316 = 0
                        }
                        frame "Log - Lin" {
                        }
                        frame "Lin - Log" {
                        }
                        frame "Log - log".. {
                          w321 = 1
                        }
                      }
                      n189 = property on="Igraph" class="XYGraph (strict)"("X Scale.Mapping Mode"=w314) -> ()  [unwired: 2 in, 2 out]
                      n190 = property on="Igraph" class="XYGraph (strict)"("Y Scale.Mapping Mode"=w313, "YScale.Minimum"=w313) -> ()  [unwired: 2 in, 2 out]
                    }
                  }
                  n191 = Subtract(x=w286, y=w269) -> (x-y=w268:dbl)
                  n192 = Not(x=w285) -> (.not. x?=w291:bool)
                  n193 = Greater Than 0?(x=w268) -> (x > 0?=w270:bool)
                  n194 = Format Into String(format string="%d", w268) -> (resulting string=w290:string)  [unwired: 2 in, 1 out]
                  n195 = And(x=w270, y=w291) -> (x .and. y?=w288:bool)
                  n196 = Concatenate Strings(w274, "\r\n", "Timer status: ", w290) -> (w284:string)
                  n197 = local write "STATUS 1"(w284) -> ()
                }
              }
              frame #1 {
                n198 = local read "abort"() -> (w323:bool)
                n199 = case shown="False" w323 {
                  tunnel: [w334 w466] -> w324
                  tunnel: w325 -> [w333 _]
                  tunnel: w326 -> [w332 _]
                  tunnel: [w330 w466] -> w327
                  tunnel: w328 -> [w331 _]
                  tunnel: [w329 w466] -> w322
                  frame False {
                    n200 = stacked-sequence {
                      seq-local: [w348 _ _] -> [_ w377 _]
                      seq-local: [w343 _ _] -> [_ _ w435]
                      tunnel: w331 -> [_ _ w440]
                      tunnel: w332 -> [_ _ w433]
                      tunnel: [_ _ w438] -> w334
                      tunnel: [_ _ w437] -> w330
                      tunnel: w333 -> [_ _ _]
                      tunnel: [w352 _ _] -> w329
                      frame #0 {
                        w346 = T3."Add Element" ("Action")
                        # "SMU data"
                        n201 = Get Date/Time String(want seconds? (F)=TRUE) -> (time string=w349:string)  [unwired: 2 in, 1 out]
                        n202 = local write "Last reading at:"(w349) -> ()
                        n203 = local write "STATUS 1"("Reading current ..." ("status")) -> ()
                        n204 = global read "QC_MeasurementSetup.vi" "GCD Measurement Parameters"() -> (w342:T6)
                        n205 = Unbundle By Name(w342) -> ("Bias Supply"=w336:refnum<class "SupplyControl.lvclass">, "Set Current Limit?"=w341:bool, "Current Limit [µA]"=w338:dbl, "Temperature Readout"=w340:enum16{"Read Arduino", "Enter manually"}, "Arduino"=w335:refnum<class "ArduinoControl.lvclass">)
                        n206 = local read "Current reading No."() -> (w345:u32)
                        n207 = local read "Current Volts:"() -> (w354:dbl)
                        n208 = case shown="\"Read Arduino\"" w340 {
                          tunnel: [w362 w368] -> w350
                          tunnel: [w359 w367] -> w344
                          tunnel: w335 -> [_ w366]
                          frame "Enter manually", Default {
                            n209 = local read "Temp."() -> (w364:dbl[])
                            n210 = local read "RH"() -> (w360:dbl[])
                            n211 = Index Array(array=w364, index=0) -> (element=w362:dbl)
                            n212 = Index Array(array=w360, index=0) -> (element=w359:dbl)
                          }
                          frame "Read Arduino" {
                            n213 = call "ArduinoRead.vi"("Arduino function"=enum16{"T/RH", "Interlock", "Edgesense"}."T/RH", "ArduinoControl in"=w366) -> ("rel. Humidity [%]"=w367:dbl, "Temperature [°C]"=w368:dbl)  [unwired: 4 in, 4 out]
                          }
                        }
                        n214 = Multiply(x=w338, y=1000.0) -> (x*y=w337:dbl)
                        n215 = call-dynamic "Supply_ReadCurrent.vi"("SupplyControl in"=w336) -> ("error out"=w343:errorcluster, "Current in nA"=w353:dbl)  [unwired: 8 in, 1 out]
                        n216 = case shown="True" w341 {
                          tunnel: w353 -> [_ w373]
                          tunnel: w337 -> [_ w371]
                          tunnel: [FALSE w370] -> w352
                          frame False {
                          }
                          frame True {
                            n217 = Absolute Value(x=w373) -> (abs(x)=w372:dbl)
                            n218 = Greater?(x=w372, y=w371) -> (0:w370:bool)
                          }
                        }
                        n219 = Increment(x=w345) -> (x+1=w348:u32)
                        n220 = call "GCDData.vi"("Action"=w346, "Array No."=u32 1, "Data IN"=w353) -> ()  [unwired: 2 in, 2 out]
                        n221 = call "GCDData.vi"("Action"=w346, "Array No."=0, "Data IN"=w354) -> ()  [unwired: 2 in, 2 out]
                        n222 = local write "Current reading No."(w348) -> ()
                        n223 = call "GCDData.vi"("Action"=w346, "Array No."=u32 2, "Data IN"=w350) -> ()  [unwired: 2 in, 2 out]
                        n224 = call "GCDData.vi"("Action"=w346, "Array No."=u32 3, "Data IN"=w344) -> ()  [unwired: 2 in, 2 out]
                      }
                      frame #1 {
                        w375 = T3."Read Array" ("Action")
                        w387 = u32 3 ("y")
                        # "Update plots"
                        n225 = property on="Igraph" class="XYGraph (strict)"() -> ("YScale.Mapping Mode"=w378:u8)  [unwired: 2 in, 2 out]
                        n226 = property on="Igraph" class="XYGraph (strict)"("YScale.Minimum"=w378) -> ()  [unwired: 2 in, 2 out]
                        n227 = call "GCDData.vi"("Action"=w375, "Array No."=1) -> ("Array OUT"=w389:dbl[])  [unwired: 3 in, 1 out]
                        n228 = Greater?(x=w377, y=w387) -> (0:w386:bool)
                        n229 = case shown="False" w386 {
                          tunnel: w377 -> [w393 w396]
                          tunnel: w387 -> [_ w395]
                          tunnel: [w393 w395] -> w385
                          tunnel: [0 w394] -> w383
                          frame False {
                          }
                          frame True {
                            n230 = Subtract(x=w396, y=w395) -> (x-y=w394:u32)
                          }
                        }
                        n231 = Array Subset(array=w389, index=0, length=w377) -> (w382:dbl[])
                        n232 = local read "Iscale"() -> (w388:enum16{"nanoAmps", "microAmps", "milliAmps"})
                        n233 = Absolute Value(x=w382) -> (abs(x)=w381:dbl[])
                        n234 = case shown="..\"nanoAmps\"" w388 {
                          tunnel: [w421 w422 w425] -> w391
                          tunnel: w381 -> [w421 w424 w427]
                          frame .."nanoAmps" {
                          }
                          frame "microAmps" {
                            n235 = Divide(x=w424, y=1000.0) -> (x/y=w422:dbl[])
                          }
                          frame "milliAmps".. {
                            n236 = Divide(x=w427, y=1000000.0) -> (x/y=w425:dbl[])
                          }
                        }
                        n237 = for {
                          N: 4 -> [_]
                          tunnel: w385 -> [w401]
                          tunnel: w383 -> [w400]
                          tunnel: w377 -> [w397]
                          i -> [w402]
                          n238 = call "GCDData.vi"("Action"=T3."Read Array", "Array No."=w402) -> ("Array OUT"=w399:dbl[])  [unwired: 3 in, 1 out]
                          n239 = case shown="..0" w402 {
                            tunnel: w401 -> [w405 w409 _ _]
                            tunnel: w400 -> [w406 w410 _ _]
                            tunnel: w399 -> [w404 w408 w414 w419]
                            tunnel: w397 -> [_ _ w412 w417]
                            frame ..0 {
                              n240 = Array Subset(array=w404, index=w406, length=w405) -> (w403:dbl[])
                              n241 = local write "Volts"(w403) -> ()
                            }
                            frame 1 {
                              n242 = Array Subset(array=w408, index=w410, length=w409) -> (w407:dbl[])
                              n243 = local write "Current"(w407) -> ()
                            }
                            frame 2 {
                              n244 = Decrement(x=w412) -> (x-1=w411:u32)
                              n245 = Array Subset(array=w414, index=w411, length=1) -> (w413:dbl[])
                              n246 = local write "Temp."(w413) -> ()
                            }
                            frame 3.. {
                              n247 = Decrement(x=w417) -> (x-1=w416:u32)
                              n248 = Array Subset(array=w419, index=w416, length=1) -> (w418:dbl[])
                              n249 = local write "RH"(w418) -> ()
                            }
                          }
                        }
                        n250 = call "GCDData.vi"("Action"=w375, "Array No."=0) -> ("Array OUT"=w374:dbl[])  [unwired: 3 in, 1 out]
                        n251 = Bundle("Array OUT"=w374, w391) -> (w379:cluster{"Array OUT":dbl[], dbl[]})  [unwired: 1 in]
                        n252 = local write "Igraph"(w379) -> ()
                      }
                      frame #2 {
                        # "Increment volts and check for end of loop"
                        n253 = local read "positive ramp?"() -> (w436:bool)
                        n254 = local read "Current Volts:"() -> (w428:dbl)
                        n255 = case shown="False" w436 {
                          tunnel: w433 -> [w443 w447]
                          tunnel: w440 -> [w444 w450]
                          tunnel: [w442 w449] -> w429
                          tunnel: [w441 w446] -> w439
                          tunnel: w428 -> [w445 w448]
                          frame False {
                            n256 = Subtract(x=w445, y=w444) -> (x-y=w441:dbl)
                            n257 = Greater Or Equal?(x=w441, y=w443) -> (x >= y?=w442:bool)
                          }
                          frame True {
                            n258 = Add(x=w448, y=w450) -> (x+y=w446:dbl)
                            n259 = Less Or Equal?(x=w446, y=w447) -> (x <= y?=w449:bool)
                          }
                        }
                        n260 = Quotient & Remainder(x=w428, y=w433) -> (x-y*floor(x/y)=w434:dbl, floor(x/y)=w432:dbl)
                        n261 = Not Equal To 0?(x=w434) -> (x != 0?=w430:bool)
                        n262 = Equal To 0?(x=w432) -> (x = 0?=w431:bool)
                        n263 = Or(x=w430, y=w431) -> ()  [unwired: 1 out]
                        n264 = case shown="True" w429 {
                          tunnel: w439 -> [_ w462]
                          tunnel: [TRUE FALSE] -> w438
                          tunnel: [FALSE w463] -> w437
                          tunnel: w428 -> [_ w460]
                          tunnel: w435 -> [_ w459]
                          frame False {
                          }
                          frame True {
                            n265 = global read "QC_MeasurementSetup.vi" "GCD Measurement Parameters"() -> (w454:T6)
                            n266 = local write "STATUS 1"("Incrementing volts.") -> ()
                            n267 = local read "step [V]"() -> (w457:dbl)
                            n268 = Unbundle By Name(w454) -> ("SMU"=w453:refnum<class "SupplyControl.lvclass">)
                            n269 = call "SupplyRamp.vi"("error in"=w459, "Requested Voltage"=w462, "Step Size"=w457, "Step Delay"=100, "Supply IN"=w453, "Starting Voltage"=w460) -> ("error out"=w455:errorcluster, "Compliance exceeded"=w463:bool, "Current Voltage"=w458:dbl)  [unwired: 2 in, 1 out]
                            n270 = case shown="No Error" w455 {
                              tunnel: w458 -> [w465 _]
                              frame No Error {
                                n271 = local write "Current Volts:"(w465) -> ()
                              }
                              frame Error {
                              }
                            }
                            n272 = property on="Bias On/Off:" class="Bool (strict)"("Blinking"=w463) -> ()  [unwired: 2 in, 2 out]
                          }
                        }
                      }
                    }
                  }
                  frame True {
                    w466 = FALSE
                  }
                }
              }
            }
            n273 = case shown="True" w243 {
              frame False {
              }
              frame True {
                n274 = property on="Bias On/Off:" class="Bool (strict)"("Blinking"=TRUE) -> ()  [unwired: 2 in, 2 out]
              }
            }
            n275 = Build Array(w244, w243, "abort", w241) -> (w248:bool[])
            n276 = Or Array Elements(Boolean array=w248) -> (logical OR=w254:bool)
            n277 = Not(x=w254) -> (.not. x?=w253:bool)
          }
        }
        frame True {
          w468 = FALSE
          # "compliance was exceeded when first voltage applied."
          # "Flag compliance as reason for end of run"
          n278 = local write "STATUS 1"("Run aborted - compliance exceeded.") -> ()
          n279 = Build Array(w468, TRUE, w468, w468) -> (w469:bool[])
        }
      }
      n280 = Search 1D Array(1D array=w231, element=TRUE) -> (index of element=w229:i32)  [unwired: 1 in]
      n281 = Increment(x=w229) -> (x+1=w228:i32)
      n282 = case shown="2" w228 {
        tunnel: ["" "Run ended normally" "Compliance exceeded" "Run aborted - by user" "Run aborted - Ilimit exceeded"] -> w223
        frame ..0 {
        }
        frame 1 {
        }
        frame 2 {
          # "Determine reason for end of run."
        }
        frame 3 {
        }
        frame 4.. {
        }
      }
      n283 = global read "QC_RunInformation.vi" "Run info"() -> (w227:T5)
      n284 = Bundle By Name(cluster=w227, "End of Run comment:"=w223) -> (w222:T5)
      n285 = global write "QC_RunInformation.vi" "Run info"(w222) -> ()
      n286 = Concatenate Strings(w223, "\r\n", "RAMPING DOWN VOLTS") -> (w226:string)
      n287 = local write "STATUS 1"(w226) -> ()
    }
    frame #4 {
      # "Ramp down and switch off supply"
      n288 = stacked-sequence {
        frame #0 {
          # "Tie up loose ends. Set volts to zero and switch to standby"
          # "Ramp down volts now"
          n289 = global read "QC_MeasurementSetup.vi" "GCD Measurement Parameters"() -> (w477:T6)
          n290 = Unbundle By Name(w477) -> ("Bias Supply"=w474:refnum<class "SupplyControl.lvclass">, "Ramp down steps [V]"=w476:dbl, "Ramp down Interval [s]"=w475:i32)
          n291 = Multiply(x=w475, y=1000) -> (x*y=w479:i32)
          n292 = local read "Bias volts [V]"() -> (w481:dbl)
          n293 = call "SupplyRamp.vi"("Requested Voltage"=0.0, "Step Size"=w476, "Step Delay"=w479, "Supply IN"=w474, "Starting Voltage"=w481) -> ("error out"=w473:errorcluster, "Supply OUT"=w472:refnum<class "SupplyControl.lvclass">)  [unwired: 3 in, 2 out]
          n294 = call-dynamic "Supply_Stby.vi"("error in (no error)"=w473, "SupplyControl in"=w472) -> ()  [unwired: 8 in, 2 out]
        }
        frame #1 {
          # "Tie up loose ends. Set volts to zero and switch to standby"
          # "Ramp down volts now"
          n295 = global read "QC_MeasurementSetup.vi" "GCD Measurement Parameters"() -> (w487:T6)
          n296 = Unbundle By Name(w487) -> ("SMU"=w484:refnum<class "SupplyControl.lvclass">, "Ramp down steps [V]"=w486:dbl, "Ramp down Interval [s]"=w485:i32)
          n297 = Multiply(x=w485, y=1000) -> (x*y=w489:i32)
          n298 = local read "Current Volts:"() -> (w492:dbl)
          n299 = call "SupplyRamp.vi"("Requested Voltage"=0.0, "Step Size"=w486, "Step Delay"=w489, "Supply IN"=w484, "Starting Voltage"=w492) -> ("error out"=w483:errorcluster, "Supply OUT"=w482:refnum<class "SupplyControl.lvclass">, "Current Voltage"=w490:dbl)  [unwired: 3 in, 1 out]
          n300 = call-dynamic "Supply_Stby.vi"("error in (no error)"=w483, "SupplyControl in"=w482) -> ()  [unwired: 8 in, 2 out]
          n301 = local write "Current Volts:"(w490) -> ()
        }
        frame #2 {
          w497 = 0
          n302 = local write "Bias On/Off:"(FALSE ("Visible")) -> ()
          n303 = local write "Current Volts:"(0.0 ("Current Volts:")) -> ()
          n304 = property on="Quit & Save" class="Bool"("DisabledEnum"=w497) -> ()  [unwired: 2 in, 2 out]
          n305 = property on="quit (no save)" class="Bool"("DisabledEnum"=w497) -> ()  [unwired: 2 in, 2 out]
          n306 = property on="abort" class="Bool (strict)"("DisabledEnum"=2) -> ()  [unwired: 2 in, 2 out]
          n307 = local write "STATUS 1"("Run finished. \nSave data?" ("STATUS 1")) -> ()
        }
        frame #3 {
          n308 = Current VI's Path() -> (path=w499:path)
          n309 = call "SaveJPEG.vi"("Test"="GCD", "File Path Control"=w499) -> ()  [unwired: 1 in, 2 out]
        }
      }
    }
    frame #5 {
      # "Loop and await decision on whether to save or junk data"
      # "Display and save data"
      n310 = local read "Scales"() -> (w511:T1)
      n311 = local read "Iscale"() -> (w510:enum16{"nanoAmps", "microAmps", "milliAmps"})
      n312 = while {
        shift-left: w510 -> [w550]
        shift-right: [w549] -> _
        shift-left: w511 -> [w552]
        shift-right: [w551] -> _
        tunnel: ["Quit & Save"] -> w513
        tunnel: ["quit (no save)"] -> w512
        stop <- w547 continue-if-true
        n313 = local read "Scales"() -> (w551:T1)
        n314 = local read "Iscale"() -> (w549:enum16{"nanoAmps", "microAmps", "milliAmps"})
        n315 = Not Equal?(x=w552, y=w551) -> (x != y?=w545:bool)
        n316 = Not Equal?(x=w550, y=w549) -> (x != y?=w544:bool)
        n317 = case shown="True" w545 {
          tunnel: w551 -> [_ w576]
          frame False {
          }
          frame True {
            n318 = case shown="..\"Lin - Lin\"" w576 {
              tunnel: [w577 1 0 w582] -> w575
              tunnel: [w577 0 1 w582] -> w574
              frame .."Lin - Lin" {
                w577 = 0
              }
              frame "Log - Lin" {
              }
              frame "Lin - Log" {
              }
              frame "Log - log".. {
                w582 = 1
              }
            }
            n319 = property on="Igraph" class="XYGraph (strict)"("X Scale.Mapping Mode"=w575) -> ()  [unwired: 2 in, 2 out]
            n320 = property on="Igraph" class="XYGraph (strict)"("Y Scale.Mapping Mode"=w574, "YScale.Minimum"=w574) -> ()  [unwired: 2 in, 2 out]
          }
        }
        n321 = case shown="True" w544 {
          tunnel: w549 -> [_ w562]
          frame False {
          }
          frame True {
            w555 = T3."Read Array" ("Action")
            n322 = property on="Igraph" class="XYGraph (strict)"() -> ("YScale.Mapping Mode"=w558:u8)  [unwired: 2 in, 2 out]
            n323 = global read "QC_MeasurementSetup.vi" "GCD Measurement Parameters"() -> (w557:T6)
            n324 = property on="Igraph" class="XYGraph (strict)"("YScale.Minimum"=w558) -> ()  [unwired: 2 in, 2 out]
            n325 = Unbundle By Name(w557) -> ("Number Of Steps"=w554:u32)
            n326 = call "GCDData.vi"("Action"=w555, "Array No."=u32 1 ("Action")) -> ("Array OUT"=w564:dbl[])  [unwired: 3 in, 1 out]
            n327 = Array Subset(array=w564, index=0, length=w554) -> (w561:dbl[])
            n328 = Absolute Value(x=w561) -> (abs(x)=w560:dbl[])
            n329 = case shown="\"microAmps\"" w562 {
              tunnel: [w567 w568 w572] -> w566
              tunnel: w560 -> [w567 w570 w573]
              frame .."nanoAmps" {
              }
              frame "microAmps" {
                n330 = Divide(x=w570, y=1000.0) -> (x/y=w568:dbl[])
              }
              frame "milliAmps".. {
                n331 = Divide(x=w573, y=1000000.0) -> (x/y=w572:dbl[])
              }
            }
            n332 = call "GCDData.vi"("Action"=w555, "Array No."=u32 0 ("Action")) -> ("Array OUT"=w553:dbl[])  [unwired: 3 in, 1 out]
            n333 = Bundle("Array OUT"=w553, w566) -> (w563:cluster{"Array OUT":dbl[], dbl[]})  [unwired: 1 in]
            n334 = local write "Igraph"(w563) -> ()
          }
        }
        n335 = local read "Run uninterrupted?"() -> (w543:bool)
        n336 = Compound Arithmetic op=OR("Quit & Save", "quit (no save)", w543) -> (invert w547:bool)
      }
      n337 = global read "QC_MeasurementSetup.vi" "GCD Measurement Parameters"() -> (w509:T6)
      n338 = Unbundle By Name(w509) -> ("Temperature Readout"=w508:enum16{"Read Arduino", "Enter manually"}, "Arduino"=w502:refnum<class "ArduinoControl.lvclass">)
      n339 = case shown="\"Read Arduino\"" w508 {
        tunnel: w502 -> [_ w542]
        frame "Enter manually", Default {
        }
        frame "Read Arduino" {
          n340 = call "ArduinoClose.vi"("ArduinoControl in"=w542) -> ()  [unwired: 9 in, 2 out]
        }
      }
      n341 = case shown="True" w512 {
        tunnel: [FALSE w584] -> w514
        frame False {
        }
        frame True {
          n342 = Two Button Dialog(message="Are you sure you don't want to save the data?", 1:"Quit" ("F button name (\"Cancel\")"), 2:"Save data" ("T button name (\"OK\")")) -> (T button?=w584:bool)
        }
      }
      n343 = local read "Run uninterrupted?"() -> (w500:bool)
      n344 = Compound Arithmetic op=OR(w513, w514, w500) -> (w507:bool)
      n345 = flat-sequence {
        tunnel: w507 -> [w518]
        tunnel: [w518] -> w503
        tunnel: [TRUE] -> w501
        tunnel: w500 -> [w516]
        frame #0 {
          n346 = case shown="True" w518 {
            tunnel: ["" w541] -> w521
            tunnel: [_ w526] -> w520
            tunnel: w516 -> [_ w523]
            frame False {
            }
            frame True {
              w537 = T3."Read Array" ("Action")
              n347 = local write "STATUS 1"("Saving Data ...") -> ()
              n348 = call "GCDData.vi"("Action"=w537, "Array No."=u32 0 ("Action")) -> ("Array OUT"=w532:dbl[])  [unwired: 3 in, 1 out]
              n349 = call "GCDData.vi"("Action"=w537, "Array No."=u32 1 ("Action")) -> ("Array OUT"=w531:dbl[])  [unwired: 3 in, 1 out]
              n350 = call "GCDData.vi"("Action"=w537, "Array No."=u32 3 ("Action")) -> ("Array OUT"=w539:dbl[])  [unwired: 3 in, 1 out]
              n351 = call "GCDData.vi"("Action"=w537, "Array No."=u32 2 ("Action")) -> ("Array OUT"=w538:dbl[])  [unwired: 3 in, 1 out]
              n352 = Build Array(w532, w531) -> (w530:dbl[][])
              n353 = call <vilib>:"Std Deviation and Variance.vi"("X"=w539) -> ("mean"=w527:dbl)  [unwired: 1 in, 2 out]
              n354 = call <vilib>:"Std Deviation and Variance.vi"("X"=w538) -> ("mean"=w528:dbl)  [unwired: 1 in, 2 out]
              n355 = Transpose 2D Array(2D array=w530) -> ()  [unwired: 1 out]
              n356 = call "SaveDataFile.vi"("Temperature"=w528, "Run uninterrupted?"=w523, "Humidity"=w527, "Array Titles"="Gate_Voltage[V] Diode_Current[nA]", "Strip Segment"="", "Arrays format"="%010.6f") -> ("Path + Filename OUT"=w541:string, "Error Out"=w526:errorcluster)  [unwired: 6 in, 2 out]
            }
          }
          n357 = call "WriteLogFile.vi"("Run uninterrupted?"=w516, "Automatic warning"="", "Data File"=w521, "Error In"=w520, "DUT passed?"=TRUE, "Files saved?"=w518) -> ()  [unwired: 5 in, 1 out]
        }
      }
      n358 = Select(t="Run finished.\nData saved." ("STATUS 1"), s=w503, f="Run finished.\nData not saved." ("STATUS 1")) -> (s? t:f=w506:string)
      n359 = local write "STATUS 1"(w506) -> ()
      "Done!" <- w501
    }
  }
